vi "Create Instrument SMO Name.vi"(8 "error in (no error)":errorcluster, 11 "Instrument.Example in":refnum<class "Instrument.LakeShore340.lvclass">) -> (0 "error out":errorcluster, 2 "SMO Name":string, 3 "Instrument.Example out":refnum<class "Instrument.LakeShore340.lvclass">)   [LabVIEW 2016, in "Instrument.LakeShore340.lvclass"]
uses:
  Instrument.LakeShore340.lvclass
  <userlib>/LevyLab/Levylab Instruments/SMOs/Instrument/Instrument.lvclass
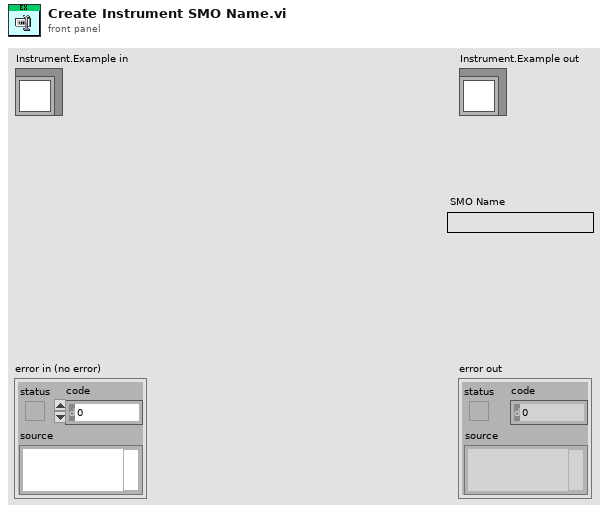
[diagram p1: front panel]
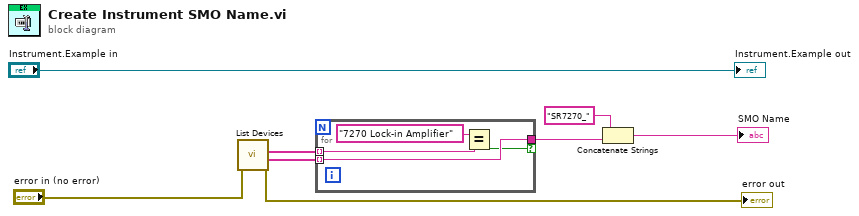
[diagram p0: block diagram]
diagram:
  n1 = call <userlib>:"List Devices.vi"("error in (no error)"="error in (no error)") -> ("error out"=→"error out":errorcluster, "Serial Numbers"=w6:string[], "Product Names"=w5:string[])  [unwired: 7 in, 1 out]
  n2 = for {
    tunnel: w5 -> [w11] mode=indexing
    tunnel: w6 -> [w10] mode=indexing
    tunnel: [w10] -> w8 if=w9
    n3 = Equal?(x="7270 Lock-in Amplifier", y=w11) -> (x = y?=w9:bool)
  }
  n4 = Concatenate Strings("SR7270_", w8) -> (→"SMO Name":string)
  "Instrument.Example out" <- "Instrument.Example in"
